vi "attribute_read_string.vi"(5 "Repeated Capability":string, 7 "Attribute":T1={"Identifier"="", "Descriptive name"="", "Data Type"=enum."Integer 32", "Command"="", "Access"=2, "Range Table"="", "Read Callback"="", "Write Callback"="", "Range Callback"="", "Check Callback"="", "Rngtable Callback"="", "Coerce Callback"="", "Supported Models"="", "Instrument Options"="", "Repeated Capabilities"="", "Check Status Callback"="", "Index"=0, "Flag: OPC Wait"=FALSE, "Flag: Dont check status"=FALSE, "Flag: Cache Only"=FALSE} {"Access" items=["Read Only", "Write Only", "Read/Write"]}, 8 "error in":errorcluster, 11 "VISA resource name":refnum<visa-resource-name>) -> (0 "error out":errorcluster, 2 "string out":string, 3 "VISA resource name out":refnum<visa-resource-name>)   [LabVIEW 2014, in "rszvl_rsidr_core.lvlib"]
uses:
  rszvl_rsidr_core.lvlib
  type_Attribute.ctl
  type_Attribute_Data_Type.ctl
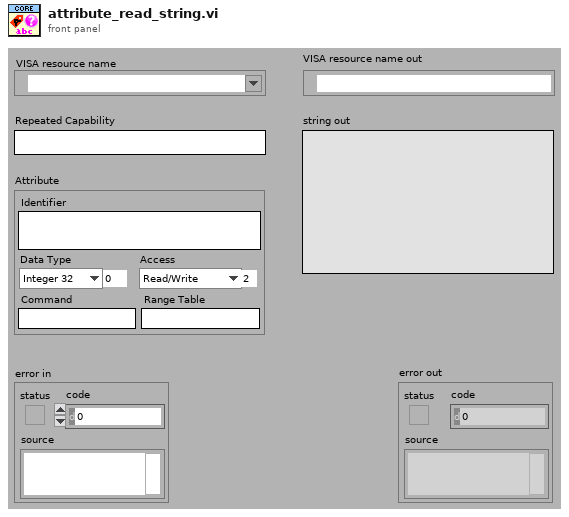
[diagram p1: front panel]
types:
  T1 = typedef "rszvl_rsidr_core.lvlib/type_Attribute.ctl" = cluster{"Identifier":string, "Descriptive name":string, "Data Type":T2, "Command":string, "Access":u16, "Range Table":string, "Read Callback":string, "Write Callback":string, "Range Callback":string, "Check Callback":string, "Rngtable Callback":string, "Coerce Callback":string, "Supported Models":string, "Instrument Options":string, "Repeated Capabilities":string, "Check Status Callback":string, "Index":i32, "Flag: OPC Wait":bool, "Flag: Dont check status":bool, "Flag: Cache Only":bool}
  T2 = typedef "rszvl_rsidr_core.lvlib/type_Attribute_Data_Type.ctl" = enum16{"Integer 32", "Double", "String", "Boolean", "None", "Integer 64"}
  T3 = typedef "rszvl_rsidr_core.lvlib/type_Session_Data.ctl" = cluster{"Instr type":string, "Instr type for err. msg.":string, "Installed Options":string[], "OPC Timeout":i32, "Query Instrument Status":bool, "Check Range":bool, "Check Options":bool, "Add LF to Write":bool, "Simulate":bool, "Logging":bool, "Logging params":variant, "Interface Type":enum16{"Unknown", "GPIB", "VXI", "GPIB_VXI", "ASRL", "PXI", "TCPIP", "USB", "SOCKET"}, "Fast Sweep":i32, "AdditionalFlags":i32, "WaitBeforeWrite":i32, "WaitBeforeRead":i32, "BinDataChunkSize":i64}
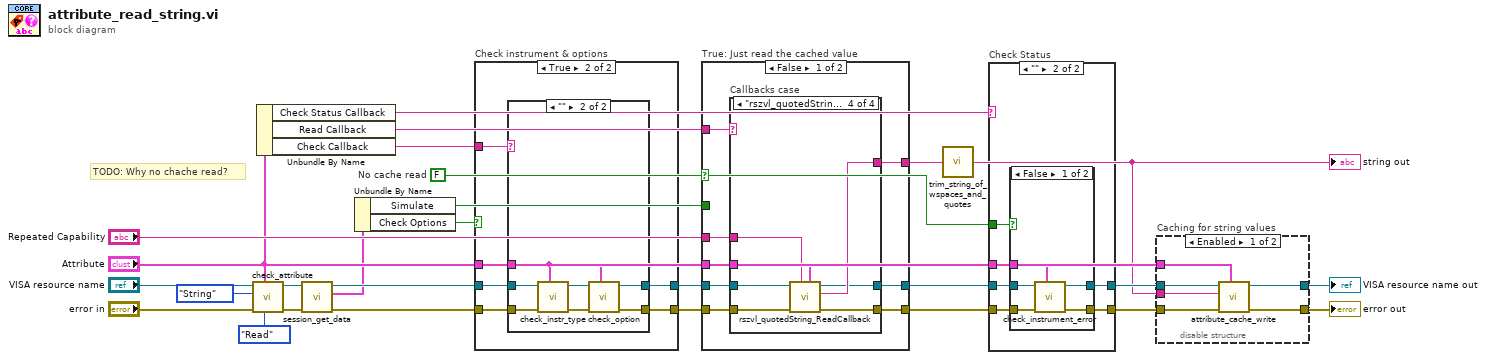
[diagram p0: block diagram]
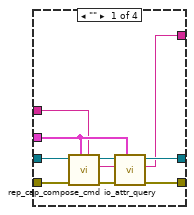
[diagram p2: hidden frame]
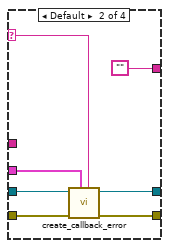
[diagram p3: hidden frame]
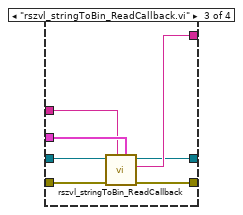
[diagram p4: hidden frame]
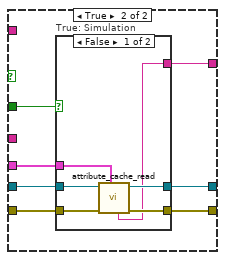
[diagram p5: hidden frame]
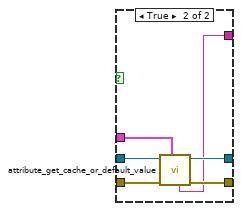
[diagram p6: hidden frame]
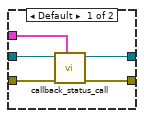
[diagram p7: hidden frame]
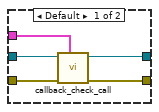
[diagram p10: hidden frame]
diagram:
  w10 = FALSE  # No cache read
  # "TODO: Why no chache read?"
  n1 = call "check_attribute.vi"("Access"=enum16{"Read", "Write"}."Read", "Attribute"="Attribute", "error in"="error in", "Data Type"=type_Attribute_Data_Type."String", "VISA resource name"="VISA resource name") -> ("error out"=w14:errorcluster, "VISA resource name out"=w15:refnum<visa-resource-name>)  [unwired: 5 in]
  n2 = Unbundle By Name("Attribute") -> ("Check Status Callback"=w16:string, "Read Callback"=w17:string, "Check Callback"=w9:string)
  n3 = call "session_get_data.vi"("error in"=w14, "VISA resource name"=w15) -> ("error out"=w13:errorcluster, "Session User Data out"=w3:T3, "VISA resource name out"=w12:refnum<visa-resource-name>)  [unwired: 7 in]
  n4 = Unbundle By Name(w3) -> ("Simulate"=w4:bool, "Check Options"=w11:bool)
  n5 = case "Check instrument & options" shown="True" w11 {
    tunnel: [w29 w35] -> w7
    tunnel: [w28 w34] -> w6
    tunnel: w9 -> [_ w33]
    tunnel: w13 -> [w28 w32]
    tunnel: w12 -> [w29 w31]
    tunnel: "Attribute" -> [_ w30]
    frame False {
    }
    frame True {
      n6 = case shown="\"\"" w33 {
        tunnel: [w39 w45] -> w35
        tunnel: [w37 w44] -> w34
        tunnel: w32 -> [w38 w43]
        tunnel: w31 -> [w40 w42]
        tunnel: w30 -> [w36 w41]
        frame Default {
          n7 = call "callback_check_call.vi"("Attribute"=w36, "error in"=w38, "VISA resource name"=w40) -> ("error out"=w37:errorcluster, "VISA resource name out"=w39:refnum<visa-resource-name>)  [unwired: 7 in]
        }
        frame "" {
          n8 = call "check_instr_type.vi"("Attribute"=w41, "error in"=w43, "VISA resource name"=w42) -> ("error out"=w47:errorcluster, "VISA resource name out"=w46:refnum<visa-resource-name>)  [unwired: 6 in, 1 out]
          n9 = call "check_option.vi"("Attribute"=w41, "error in"=w47, "VISA resource name"=w46) -> ("error out"=w44:errorcluster, "VISA resource name out"=w45:refnum<visa-resource-name>)  [unwired: 7 in]
        }
      }
    }
  }
  n10 = case "True: Just read the cached value" shown="False" w10 {
    tunnel: "Repeated Capability" -> [w55 _]
    tunnel: [w54 w89] -> w19
    tunnel: [w53 w90] -> w18
    tunnel: [w52 w88] -> w2
    tunnel: w17 -> [w51 _]
    tunnel: w7 -> [w50 w93]
    tunnel: w6 -> [w49 w91]
    tunnel: "Attribute" -> [w48 w92]
    tunnel: w4 -> [_ w87]
    frame False {
      n11 = case "Callbacks case" shown="\"rszvl_quotedString_ReadCallback.vi\"" w51 {
        selector: w51 -> [_ w68 _ _]
        tunnel: w50 -> [w65 w71 w78 w85]
        tunnel: w49 -> [w64 w72 w79 w86]
        tunnel: w55 -> [w57 _ w76 w83]
        tunnel: [w63 w69 w73 w80] -> w53
        tunnel: [w62 w70 w74 w81] -> w54
        tunnel: [w56 "" ("Empty String Constant") w75 w82] -> w52
        tunnel: w48 -> [w58 w67 w77 w84]
        frame "" {
          n12 = call "rep_cap_compose_cmd.vi"("Repeated Capability"=w57, "Attribute"=w58, "error in"=w64, "VISA resource name"=w65) -> ("error out"=w61:errorcluster, "Command out"=w60:string, "VISA resource name out"=w59:refnum<visa-resource-name>)  [unwired: 5 in]
          n13 = call "io_attr_query.vi"("Attribute"=w58, "error in"=w61, "write buffer"=w60, "VISA resource name"=w59) -> ("error out"=w62:errorcluster, "read buffer"=w56:string, "VISA resource name out"=w63:refnum<visa-resource-name>)  [unwired: 5 in]
        }
        frame Default {
          n14 = call "create_callback_error.vi"("Callback Name"=w68, "Attribute"=w67, "error in"=w72, "VISA resource name"=w71) -> ("error out"=w70:errorcluster, "VISA resource name out"=w69:refnum<visa-resource-name>)  [unwired: 6 in]
        }
        frame "rszvl_stringToBin_ReadCallback.vi" {
          n15 = call "rszvl_stringToBin_ReadCallback.vi"("Attribute"=w77, "Repeated Capability"=w76, "error in"=w79, "VISA resource name"=w78) -> ("error out"=w74:errorcluster, "Attribute Value String"=w75:string, "VISA resource name out"=w73:refnum<visa-resource-name>)  [unwired: 5 in]
        }
        frame "rszvl_quotedString_ReadCallback.vi" {
          n16 = call "rszvl_quotedString_ReadCallback.vi"("Attribute"=w84, "Repeated Capability"=w83, "error in"=w86, "VISA resource name"=w85) -> ("error out"=w81:errorcluster, "Attribute Value String"=w82:string, "VISA resource name out"=w80:refnum<visa-resource-name>)  [unwired: 5 in]
        }
      }
    }
    frame True {
      n17 = case "True: Simulation" shown="False" w87 {
        tunnel: w91 -> [w99 w105]
        tunnel: w93 -> [w98 w104]
        tunnel: w92 -> [w97 w101]
        tunnel: [w96 w103] -> w89
        tunnel: [w95 w102] -> w90
        tunnel: [w94 w100] -> w88
        frame False {
          n18 = call "attribute_cache_read.vi"("Attribute"=w97, "error in"=w99, "VISA resource name"=w98) -> ("error out"=w96:errorcluster, "VISA resource name out"=w95:refnum<visa-resource-name>, "String out"=w94:string)  [unwired: 1 in, 5 out]
        }
        frame True {
          n19 = call "attribute_get_cache_or_default_value.vi"("Attribute"=w101, "error in"=w105, "VISA resource name"=w104) -> ("error out"=w103:errorcluster, "VISA resource name out"=w102:refnum<visa-resource-name>, "String out"=w100:string)  [unwired: 1 in, 5 out]
        }
      }
    }
  }
  n20 = call "trim_string_of_wspaces_and_quotes.vi"("String in"=w2) -> ("String out"=w1:string)  [unwired: 4 in]
  "string out" <- w1
  n21 = case "Check Status" shown="\"\"" w16 {
    tunnel: w19 -> [w110 w114]
    tunnel: [w109 w113] -> w23
    tunnel: [w108 w115] -> w24
    tunnel: w18 -> [w107 w116]
    tunnel: "Attribute" -> [w106 w112]
    tunnel: w10 -> [_ w111]
    frame Default {
      n22 = call "callback_status_call.vi"("Attribute"=w106, "error in"=w110, "VISA resource name"=w107) -> ("error out"=w109:errorcluster, "VISA resource name out"=w108:refnum<visa-resource-name>)  [unwired: 7 in]
    }
    frame "" {
      n23 = case shown="False" w111 {
        tunnel: w116 -> [w121 w123]
        tunnel: [w120 w123] -> w115
        tunnel: w114 -> [w119 w122]
        tunnel: [w118 w122] -> w113
        tunnel: w112 -> [w117 _]
        frame False {
          n24 = call "check_instrument_error.vi"("Attribute"=w117, "error in"=w119, "VISA resource name"=w121) -> ("error out"=w118:errorcluster, "VISA resource name out"=w120:refnum<visa-resource-name>)  [unwired: 7 in]
        }
        frame True {
        }
      }
    }
  }
  n25 = disable-structure "Caching for string values" shown="Enabled" {
    disable-tunnel: [w129 w131] -> w22
    disable-tunnel: [w128 w130] -> w21
    disable-tunnel: w23 -> [w127 w130]
    disable-tunnel: w24 -> [w126 w131]
    disable-tunnel: w1 -> [w125 _]
    disable-tunnel: "Attribute" -> [w124 _]
    frame Enabled {
      n26 = call "attribute_cache_write.vi"("Attribute"=w124, "error in"=w127, "Value in"=w125, "VISA resource name"=w126) -> ("error out"=w128:errorcluster, "VISA resource name out"=w129:refnum<visa-resource-name>)  [unwired: 6 in]
    }
    frame Disabled {
    }
  }
  "error out" <- w21
  "VISA resource name out" <- w22
